vi "Get Table Names SQLServer.vi"(8 "error in (no error)":errorcluster, 11 "ADODB._Connection":refnum<k7>) -> (0 "error out":errorcluster, 2 "List Of Tables":string[](array[string]), 3 "ADODB._Connection":refnum<k7>)   [LabVIEW 2017]
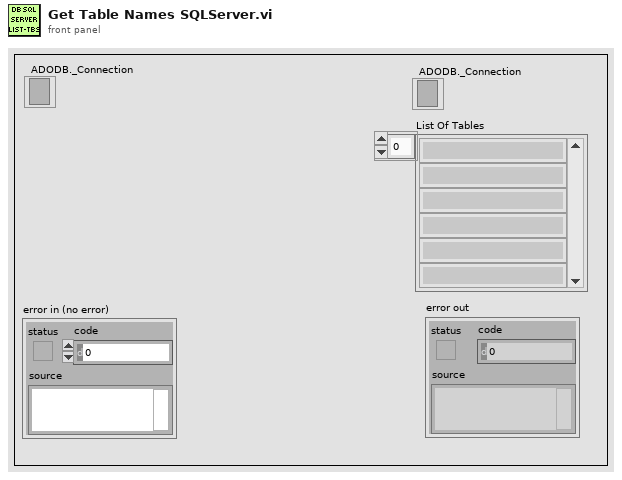
[diagram p1: front panel]
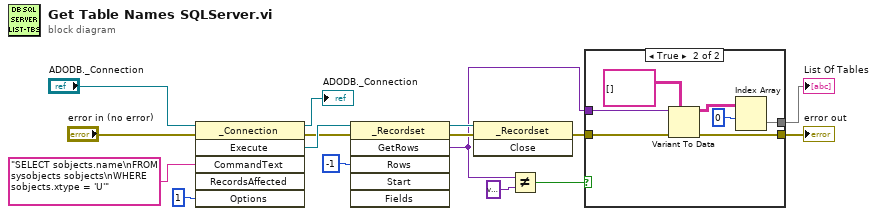
[diagram p0: block diagram]
diagram:
  n1 = invoke class="_Connection" method="Execute"(reference="ADODB._Connection", error in="error in (no error)", "CommandText"="SELECT sobjects.name\nFROM sysobjects sobjects\nWHERE sobjects.xtype = 'U'", "Options"=1) -> (reference out=→"ADODB._Connection":refnum<k7>, error out=w9:errorcluster, "Execute"=w12:refnum<k7>)  [unwired: 2 in, 3 out]
  n2 = invoke class="_Recordset" method="GetRows"(reference=w12, error in=w9, "Rows"=-1) -> (reference out=w11:refnum<k7>, error out=w8:errorcluster, "GetRows"=w5:variant)  [unwired: 3 in, 3 out]
  n3 = invoke class="_Recordset" method="Close"(reference=w11, error in=w8) -> (error out=w2:errorcluster)  [unwired: 1 in, 2 out]
  n4 = Not Equal?(x=w5, y=variant) -> (x != y?=w3:bool)
  n5 = case shown="True" w3 {
    tunnel: [_ w18] -> w7
    tunnel: w5 -> [_ w24]
    tunnel: w2 -> [w17 w23]
    tunnel: [w17 w22] -> w1
    frame False {
    }
    frame True {
      n6 = Variant To Data(error in=w23, type=string[][] [], Variant=w24) -> (data=w20:string[][], error out=w22:errorcluster)
      n7 = Index Array(array=w20, index (row)=0) -> (element=w18:string[])  [unwired: 1 in]
    }
  }
  "error out" <- w1
  "List Of Tables" <- w7
